vi "GetExternalInterfaces.vi"(8 "Error In":errorcluster, 11 "reference in":refnum<class "TemplateGUI.lvclass">) -> (0 "Error Out":errorcluster, 2 "ExternalInterfaces":T1[](array[typedef]), 3 "reference out":refnum<class "TemplateGUI.lvclass">)   [LabVIEW 2021, in "TemplateGUI.lvlib" / "TemplateGUI.lvclass"]
uses:
  TemplateGUI.lvclass
  .Externals/Library_TAF_Support/ClusterArrayConversion/BundledArray.ctl
  c918bead-a22c-460a-a6f4-f95520c4e6a6.vi
  c918bead-a22c-460a-a6f4-f95520c4e6a6.vi/e733eca7-9823-4359-8665-3b184f9a7377.vi
  <vilib>/Utility/Data Type/Get Cluster Information.vi
  <vilib>/Utility/Data Type/Get Type Information.vi
  .Externals/Library_TAF_Support/ClusterArrayConversion/ClusterArrayConversion.lvlib
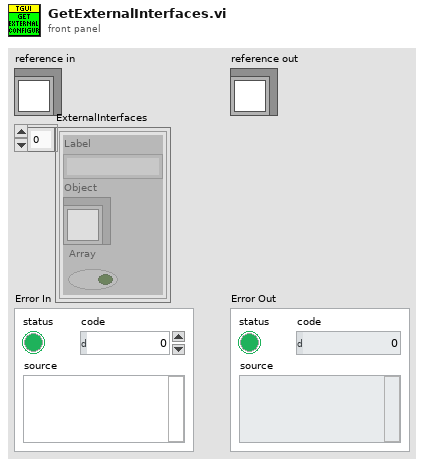
[diagram p1: front panel]
types:
  T1 = typedef "ClusterArrayConversion.lvlib/BundledArray.ctl" = cluster{"Label":string, "Object":refnum<class>, "Array":bool}
  T2 = typedef "TemplateGUI.lvlib/TemplateGUI.lvclass/ObjectAttributes.ctl" = cluster{"Interfaces":cluster{"Dummys":refnum<class>}, "Locals":cluster{"MainGUIActive":refnum<queue>}, "Persistent":cluster{"Dummy":bool}}
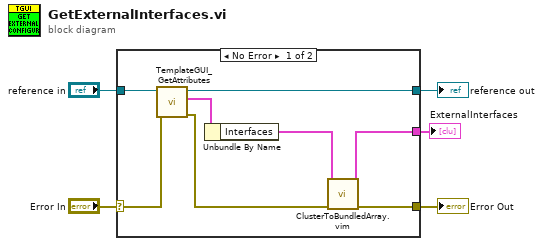
[diagram p0: block diagram]
diagram:
  n1 = case shown="No Error" "Error In" {
    selector: "Error In" -> [w13 w15]
    tunnel: [w6 w15] -> w4
    tunnel: [w10 w14] -> w2
    tunnel: "reference in" -> [w11 w14]
    tunnel: [w7 _] -> w1
    frame No Error {
      n2 = call "TemplateGUI_GetAttributes.vi"("error in (no error)"=w13, "reference in"=w11) -> ("error out"=w9:errorcluster, "Data"=w12:T2, "reference out"=w10:refnum<class "TemplateGUI.lvclass">)  [unwired: 6 in, 1 out]
      n3 = Unbundle By Name(w12) -> ("Interfaces"=w8:cluster{"Dummys":refnum<class>})
      n4 = call "ClusterToBundledArray.vim"("error in (no error)"=w9, "Interfaces"=w8) -> ("error out"=w6:errorcluster, "BundeledLabels"=w7:T1[])  [unwired: 8 in]
    }
    frame Error {
    }
  }
  "Error Out" <- w4
  "reference out" <- w2
  "ExternalInterfaces" <- w1
